vi "RestorationCaracteresInterdits.vi"(8 "error in (no error)":errorcluster, 11 "String In":string) -> (0 "error out":errorcluster, 3 "String Out":string)   [LabVIEW 2011]
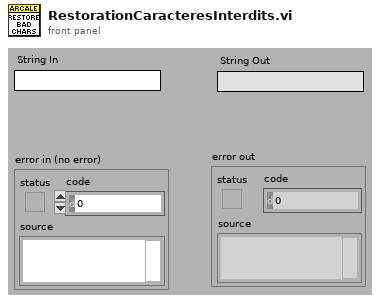
[diagram p1: front panel]
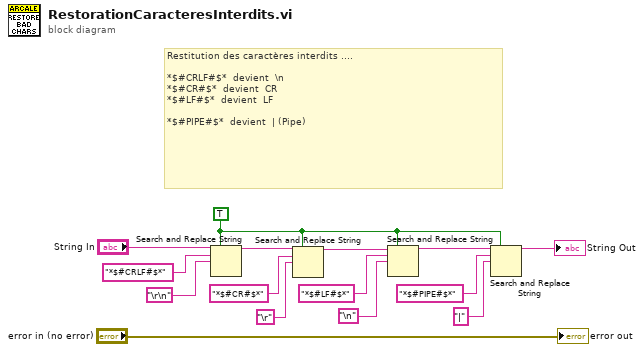
[diagram p0: block diagram]
diagram:
  w10 = TRUE ("replace all? (F)")
  # "Restitution des caractères interdits ....\n\n*$#CRLF#$*  devient  \\n \n*$#CR#$*  devient  CR\n*$#LF#$*  devient  LF\n\n*$#PIPE#$*  devient  | (Pipe)"
  n1 = Search and Replace String(replace all?=w10, input string="String In", search string="*$#CRLF#$*", replace string="\r\n") -> (result string=w14:string)  [unwired: 4 in, 3 out]
  n2 = Search and Replace String(replace all?=w10, input string=w14, search string="*$#CR#$*", replace string="\r") -> (result string=w13:string)  [unwired: 4 in, 3 out]
  n3 = Search and Replace String(replace all?=w10, input string=w13, search string="*$#LF#$*", replace string="\n") -> (result string=w11:string)  [unwired: 4 in, 3 out]
  n4 = Search and Replace String(replace all?=w10, input string=w11, search string="*$#PIPE#$*", replace string="|" ("search string")) -> (result string=→"String Out":string)  [unwired: 4 in, 3 out]
  "error out" <- "error in (no error)"
